vi "input.vi"(8 "error in (no error)":errorcluster caption="错误输入（无错误）", 10 "布尔":bool, 11 "ShopBase输入":refnum<class "ShopBase.lvclass">) -> (0 "error out":errorcluster caption="错误输出", 3 "ShopBase输出":refnum<class "ShopBase.lvclass">)   [LabVIEW 2013, in "ShopBase.lvclass"]
uses:
  ShopBase.lvclass
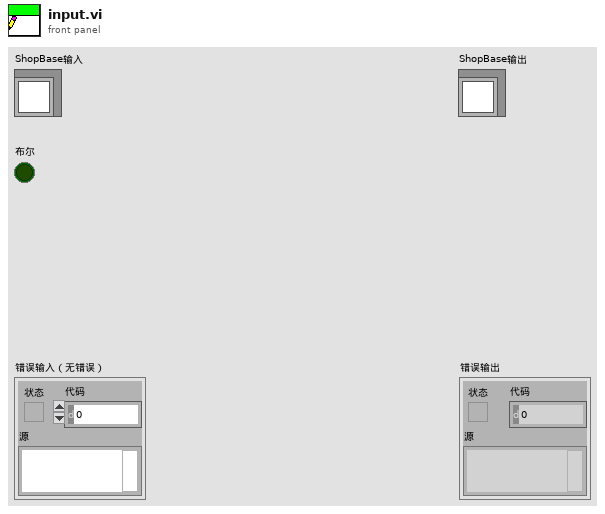
[diagram p1: front panel]
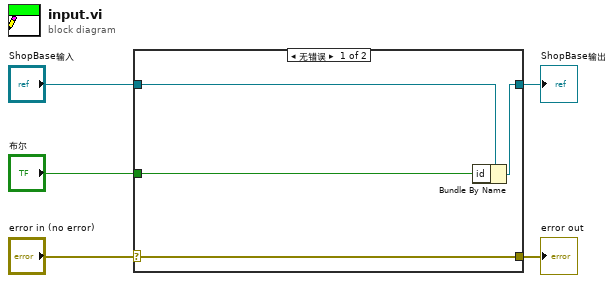
[diagram p0: block diagram]
diagram:
  n1 = case shown="无错误" "error in (no error)" {
    selector: "error in (no error)" -> [w9 w10]
    tunnel: [w9 w10] -> w4
    tunnel: [w7 w11] -> w2
    tunnel: "ShopBase输入" -> [w8 w11]
    tunnel: "布尔" -> [w6 _]
    frame No Error {
      n2 = Bundle By Name(cluster=w8, "id"=w6) -> (w7:refnum<class "ShopBase.lvclass">)
    }
    frame Error {
    }
  }
  "error out" <- w4
  "ShopBase输出" <- w2
